vi "ccdChipPixels.vi"() -> ()   [LabVIEW 2013]
panel:
  in  "CCD Chip horizontal end":i32
  in  "CCD Chip Vertical end":i32
  in  "CCD Chip horizontal start":i32
  in  "CCD Chip Vertical Start":i32
  in  "CCD Chip Size":i32
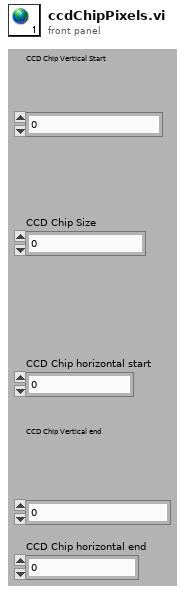
[diagram p1: front panel]
diagram:
